vi "Enque Image (Tag) (SubVI).vi"(8 "Data Bundle":T1, 11 "Tag Image REF":refnum<queue>) -> ()   [LabVIEW 2020]
uses:
  Controls (HOST)/Data to Disk Bundle.ctl
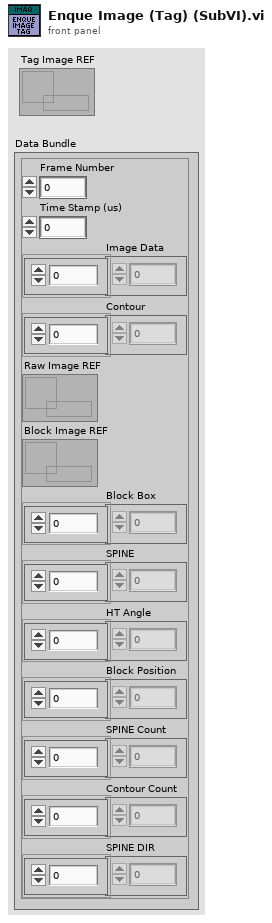
[diagram p1: front panel]
types:
  T1 = typedef "Data to Disk Bundle.ctl" = cluster{"Frame Number":u64, "Time Stamp (us)":u64, "Image Data":u64[], "Contour":u32[], "Raw Image REF":refnum<data-value>, "Block Image REF":refnum<data-value>, "Block Box":u64[], "SPINE":u32[], "HT Angle":u64[], "Block Position":u64[], "SPINE Count":u32[], "Contour Count":u32[], "SPINE DIR":u8[]}
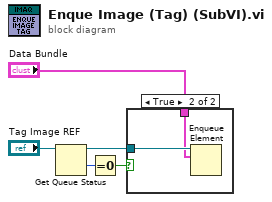
[diagram p0: block diagram]
diagram:
  n1 = Get Queue Status(queue="Tag Image REF") -> (queue out=w5:refnum<queue>, # elements in queue=w3:i32)  [unwired: 2 in, 6 out]
  n2 = Equal To 0?(x=w3) -> (x = 0?=w4:bool)
  n3 = case shown="True" w4 {
    tunnel: w5 -> [_ w7]
    tunnel: "Data Bundle" -> [_ w6]
    frame False {
    }
    frame True {
      n4 = Enqueue Element(queue=w7, element=w6) -> ()  [unwired: 2 in, 3 out]
    }
  }
